vi "Track and Move.vi"() -> ()   [LabVIEW 2012]
uses:
  <vilib>/Platform/TimedLoop/XDataNode/timing_clust.ctl
  <vilib>/Platform/TimedLoop/XDataNode/nitl_modes.ctl
  <vilib>/Platform/TimedLoop/XDataNode/wakeup.ctl
  <vilib>/robotics/Starter Kit/2.0/9632 Host Interface/NI_Robotics_Starter Kit Host_9632_2.0.lvclass
  <vilib>/Platform/TimedLoop/XDataNode/XDataNode.xnode
  <vilib>/Platform/TimedLoop/XDataNode/XDNodeRunTimeDep.lvlib
  <vilib>/robotics/Starter Kit/Host Interface/NI_Robotics_Starter Kit Host.lvclass
  <vilib>/httpClient/LabVIEWHTTPClient.lvlib
panel:
  out "file body":string
  out "Grab image error":errorcluster
  out "Vision error":errorcluster
  out "Starter kit error":errorcluster
  in  "Speed":dbl=0.25
  out "Found?":bool
  out "Right DC rad/s":dbl
  out "Left DC rad/s":dbl
  out "Angle":dbl
  out "Degrees":dbl
  out "a":dbl
  out "b":i32
  out "sign":i32
  out "speed":dbl
  out "Wz":dbl
  out "Image 2":T1(plugin-control)
  out "Image":T1(plugin-control)
  in  "stop":bool
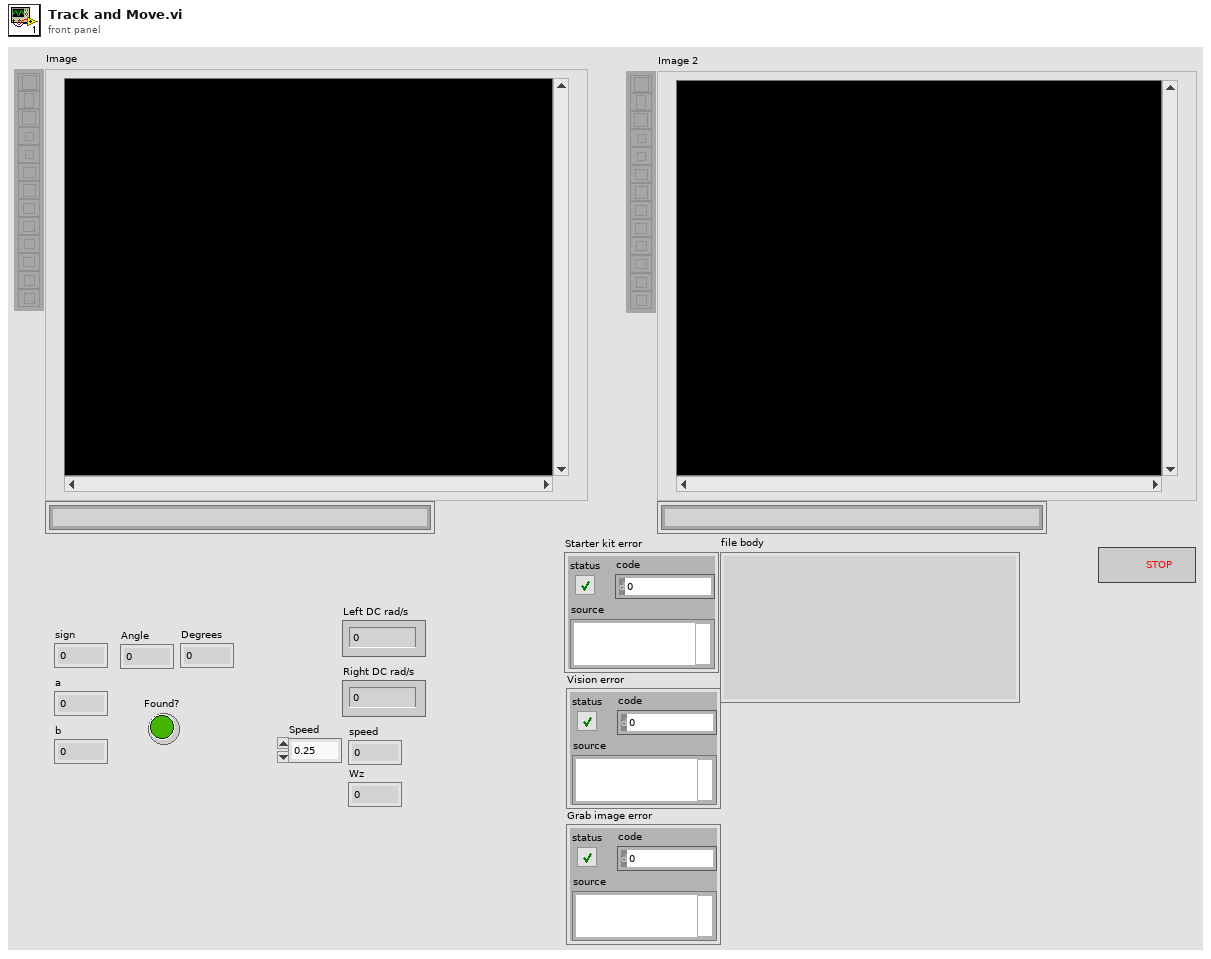
[diagram p1: front panel]
types:
  T1 = typedef "IMAQ Image.ctl" = refnum<image>
  T2 = typedef "XDNodeRunTimeDep.lvlib/timing_clust.ctl" = cluster{"Expected End [f-1]":u64, "Actual End [f-1]":u64, "Finished Late? [f-1]":bool, "Expected End [i-1]":u64, "Actual End [i-1]":u64, "Finished Late? [i-1]":bool, "Expected Start [i]":u64, "Actual Start [i]":u64, "Expected Start [f]":u64, "Actual Start [f]":u64, "Source Name":string, "Structure Name":string, "Period":i64, "Deadline":i64, "Offset":i64, "Start":i64, "Priority":i32, "Timeout":i32, "Mode":T3, "Wakeup Reason":T4, "Error":errorcluster, "Source Type":string, "Secondary Source Type":string, "Global End Time":u64, "Global Start Time":u64, "Frame Duration":u64, "Iteration Duration":u64, "Assigned CPU":i32, "I/O Scan Engine Mode":u32}
  T3 = typedef "XDNodeRunTimeDep.lvlib/nitl_modes.ctl" = enum32{"No Change", "Process missed periods, maintain original phase", "Discard missed periods, maintain original phase", "Process missed periods, ignore original phase", "Discard missed periods, ignore original phase"}
  T4 = typedef "XDNodeRunTimeDep.lvlib/wakeup.ctl" = enum32{"Normal", "Aborted", "Asynchronous wakeup", "Timing source error", "Timed loop error", "Timeout"}
  T5 = enum16{"open", "open or create", "create or replace", "create", "open (read only)"}
  T6 = typedef "Image Type" = u32
  T7 = cluster{"Global Rectangle":cluster{"x1Left":i32, "y1Top":i32, "x2Right":i32, "y2Bottom":i32}, "Centroid":cluster{"x":sgl, "y":sgl}, "Object Size":u32, "Score":dbl}[]
  T8 = cluster{"Shape Report (Shape Matching 1)[0]":cluster{"Global Rectangle":cluster{"x1Left":i32, "y1Top":i32, "x2Right":i32, "y2Bottom":i32}, "Centroid":cluster{"x":sgl, "y":sgl}, "Object Size":u32, "Score":dbl}, "Shape Report (Shape Matching 1)[1]":cluster{"Global Rectangle":cluster{"x1Left":i32, "y1Top":i32, "x2Right":i32, "y2Bottom":i32}, "Centroid":cluster{"x":sgl, "y":sgl}, "Object Size":u32, "Score":dbl}, "Shape Report (Shape Matching 1)[2]":cluster{"Global Rectangle":cluster{"x1Left":i32, "y1Top":i32, "x2Right":i32, "y2Bottom":i32}, "Centroid":cluster{"x":sgl, "y":sgl}, "Object Size":u32, "Score":dbl}, "Shape Report (Shape Matching 1)[3]":cluster{"Global Rectangle":cluster{"x1Left":i32, "y1Top":i32, "x2Right":i32, "y2Bottom":i32}, "Centroid":cluster{"x":sgl, "y":sgl}, "Object Size":u32, "Score":dbl}, "Shape Report (Shape Matching 1)[4]":cluster{"Global Rectangle":cluster{"x1Left":i32, "y1Top":i32, "x2Right":i32, "y2Bottom":i32}, "Centroid":cluster{"x":sgl, "y":sgl}, "Object Size":u32, "Score":dbl}, "Shape Report (Shape Matching 1)[5]":cluster{"Global Rectangle":cluster{"x1Left":i32, "y1Top":i32, "x2Right":i32, "y2Bottom":i32}, "Centroid":cluster{"x":sgl, "y":sgl}, "Object Size":u32, "Score":dbl}, "Shape Report (Shape Matching 1)[6]":cluster{"Global Rectangle":cluster{"x1Left":i32, "y1Top":i32, "x2Right":i32, "y2Bottom":i32}, "Centroid":cluster{"x":sgl, "y":sgl}, "Object Size":u32, "Score":dbl}, "Shape Report (Shape Matching 1)[7]":cluster{"Global Rectangle":cluster{"x1Left":i32, "y1Top":i32, "x2Right":i32, "y2Bottom":i32}, "Centroid":cluster{"x":sgl, "y":sgl}, "Object Size":u32, "Score":dbl}, "Shape Report (Shape Matching 1)[8]":cluster{"Global Rectangle":cluster{"x1Left":i32, "y1Top":i32, "x2Right":i32, "y2Bottom":i32}, "Centroid":cluster{"x":sgl, "y":sgl}, "Object Size":u32, "Score":dbl}}
  T9 = cluster{"x1Left":i32, "y1Top":i32, "x2Right":i32, "y2Bottom":i32}
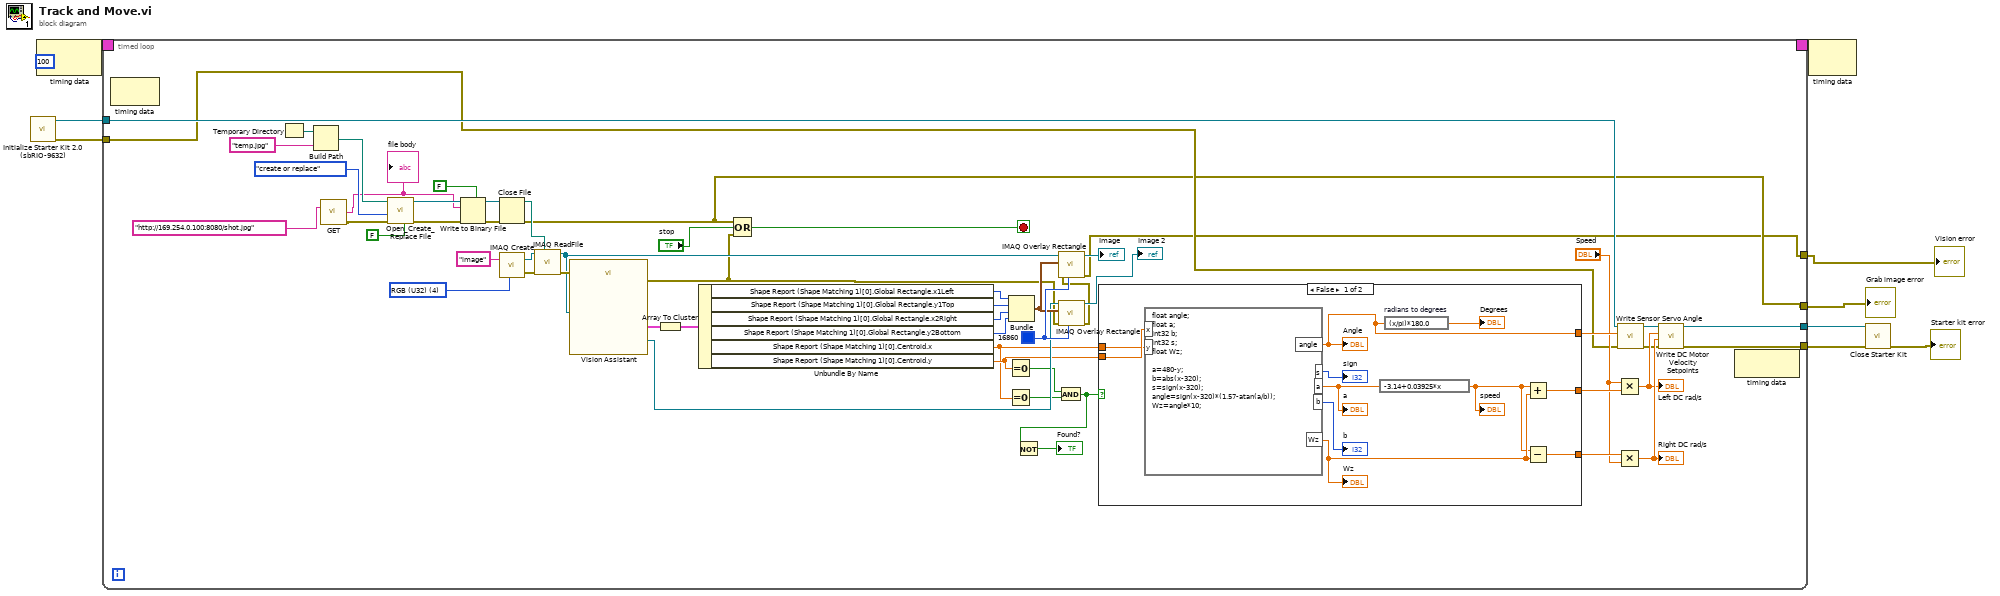
[diagram p0: block diagram]
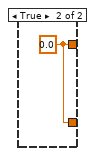
[diagram p2: hidden frame]
diagram:
  n1 = call <vilib>:"Initialize Starter Kit 2.0 (sbRIO-9632).vi"() -> ("error out"=w5:errorcluster, "FPGA starter kit host 2.0 out"=w6:refnum<class "NI_Robotics_Starter Kit Host_9632_2.0.lvclass">)  [unwired: 10 in]
  n2 = node-c288(i64 100 ("Period")) -> (w10:T2)
  n3 = timed-loop {
    timing: w10 -> [_]
    timing-out: [_] -> w9
    tunnel: [w24] -> w7
    tunnel: w6 -> [w23]
    tunnel: w5 -> [w18]
    tunnel: [w20] -> w4
    tunnel: [w17] -> w1
    tunnel: [w14] -> w2
    stop <- w39 stop-if-true
    w46 = T6 4 items=["Grayscale (U8)", "Grayscale (I16)", "Grayscale (SGL)", "Complex (CSG)", "RGB (U32)", "HSL (U32)", "RGB (U64)", "Grayscale (U16)"] ("Image Type")
    w62 = u32 16860 ("Color")
    n4 = node-c288() -> ()  [unwired: 1 in, 1 out]
    n5 = Temporary Directory() -> (w55:path)
    n6 = Build Path(base path=w55, name or relative path="temp.jpg") -> (appended path=w47:path)
    n7 = call <vilib>:"GET.vi"("url"="http://169.254.0.100:8080/shot.jpg" ("connection in")) -> ("body"=w12:string, "error out"=w11:errorcluster)  [unwired: 11 in, 2 out]
    "file body" <- w12
    n8 = call <vilib>:"Open_Create_Replace File.vi"("advisory dialog? (display:T)"=FALSE, "error in (no error)"=w11, "function (open:0)"=T5."create or replace", "file path"=w47) -> ("error out"=w52:errorcluster, "refnum"=w53:refnum<file>)  [unwired: 3 in, 3 out]
    n9 = Write to Binary File(file (use dialog)=w53, data=w12, error in=w52, 5:FALSE ("prepend array or string size? (T)")) -> (refnum out=w51:refnum<file>, error out=w50:errorcluster)  [unwired: 3 out]
    n10 = Close File(refnum=w51, error in=w50) -> (path=w43:path, error out=w17:errorcluster)
    n11 = call "IMAQ Create"("Image Name"="image", "Image Type"=w46) -> ("New Image"=w44:T1, "error out"=w37:errorcluster)  [unwired: 3 in]
    n12 = call "IMAQ ReadFile"("File Path"=w43, "error in (no error)"=w37, "Image"=w44) -> ("error out"=w38:errorcluster, "Image Out"=w36:T1)  [unwired: 4 in, 3 out]
    n13 = call "Vision Assistant"("Image In"=w36, "error in"=w38) -> ("Image Out"=w41:T1, "Shape Report (Shape Matching 1)"=w42:T7, "error out"=w16:errorcluster)  [unwired: 23 in]
    n14 = Array To Cluster(array=w42) -> (cluster=w65:T8)
    n15 = Unbundle By Name(w65) -> ("Shape Report (Shape Matching 1)[0].Global Rectangle.x1Left"=w57:i32, "Shape Report (Shape Matching 1)[0].Global Rectangle.y1Top"=w58:i32, "Shape Report (Shape Matching 1)[0].Global Rectangle.x2Right"=w59:i32, "Shape Report (Shape Matching 1)[0].Global Rectangle.y2Bottom"=w60:i32, "Shape Report (Shape Matching 1)[0].Centroid.x"=w28:sgl, "Shape Report (Shape Matching 1)[0].Centroid.y"=w29:sgl)
    n16 = Compound Arithmetic op=OR(w17, "stop", w16) -> (w39:bool)
    n17 = Equal To 0?(x=w29) -> (x = 0?=w35:bool)
    n18 = Equal To 0?(x=w28) -> (x = 0?=w34:bool)
    n19 = Bundle("x1Left"=w57, "y1Top"=w58, "x2Right"=w59, "y2Bottom"=w60) -> (w61:T9)  [unwired: 1 in]
    n20 = call "IMAQ Overlay Rectangle"("Color"=w62, "error in (no error)"=w16, "Rectangle"=w61, "Image"=w41) -> ("error out"=w15:errorcluster, "Image Out"=→"Image 2":T1)  [unwired: 6 in]
    n21 = call "IMAQ Overlay Rectangle"("Color"=w62, "error in (no error)"=w15, "Rectangle"=w61, "Image"=w36) -> ("error out"=w14:errorcluster, "Image Out"=→"Image":T1)  [unwired: 6 in]
    n22 = And(x=w35, y=w34) -> (x .and. y?=w32:bool)
    n23 = Not(x=w32) -> (.not. x?=→"Found?":bool)
    n24 = case shown="False" w32 {
      tunnel: w28 -> [w72 _]
      tunnel: w29 -> [w73 _]
      tunnel: [w70 w77] -> w31
      tunnel: [w69 w77] -> w30
      tunnel: [w66 _] -> w27
      frame False {
        n25 = formula code="float angle;\nfloat a;\nint32 b;\nint32 s;\nfloat Wz;\n\na=480-y;\nb=abs(x-320);\ns=sign(x-320);\nangle=sign(x-320)*(1.57-atan(a/b));\nWz=angle*10;"("x"=w73, "y"=w72) -> ("angle"=w66:dbl, "a"=w68:dbl, "b"=→"b":i32, "s"=→"sign":i32, "Wz"=w71:dbl)
        "Angle" <- w66
        "a" <- w68
        "Wz" <- w71
        n26 = expression code="-3.14+0.03925*x"(w68) -> (w67:dbl)
        "speed" <- w67
        n27 = expression code="(x/pi)*180.0" "radians to degrees"(w66) -> (→"Degrees":dbl)
        n28 = Add(x=w67, y=w71) -> (x+y=w70:dbl)
        n29 = Subtract(x=w67, y=w71) -> (x-y=w69:dbl)
      }
      frame True {
        w77 = 0.0
      }
    }
    n30 = Multiply(x="Speed", y=w31) -> (x*y=w25:dbl)
    "Left DC rad/s" <- w25
    n31 = Multiply(x=w30, y="Speed") -> (x*y=w26:dbl)
    "Right DC rad/s" <- w26
    n32 = call <vilib>:"Write Sensor Servo Angle.vi"("error in (no error)"=w18, "ccw servo angle (rad)"=w27, "starter kit host in"=w23) -> ("error out"=w19:errorcluster, "starter kit host out"=w22:refnum<class "NI_Robotics_Starter Kit Host_9632_2.0.lvclass">)  [unwired: 7 in]
    n33 = call <vilib>:"Write DC Motor Velocity Setpoints.vi"("error in (no error)"=w19, "right motor ccw velocity (rad/s)"=w26, "left motor ccw velocity (rad/s)"=w25, "starter kit host in"=w22) -> ("error out"=w20:errorcluster, "starter kit host out"=w24:refnum<class "NI_Robotics_Starter Kit Host_9632_2.0.lvclass">)  [unwired: 6 in]
    n34 = node-c288() -> ()  [unwired: 1 in, 1 out]
  }
  "Vision error" <- w2
  "Grab image error" <- w1
  n35 = node-c288(w9) -> ()  [unwired: 1 out]
  n36 = call-dynamic "Close Starter Kit.vi"("error in (no error)"=w4, "starter kit host in"=w7) -> ("error out"=→"Starter kit error":errorcluster)  [unwired: 9 in]
